vi "Create Framework Status.vi"(8 "error in (no error)":errorcluster, 11 "Framework Configuration":refnum<class "Framework Configuration.lvclass">) -> (0 "error out":errorcluster, 3 "Framework Status":refnum<class "Framework Status.lvclass">)   [LabVIEW 2021, in "DSF Core.lvlib" / "Framework Status.lvclass"]
uses:
  Framework Status.lvclass
  Configuration/Core/Framework/Framework Configuration.lvclass
  Status/Status Data.ctl
  <vilib>/NI/Memory Manager/Classes/Pointer/Pointer.lvclass/Pointer.ctl
  Framework Status.lvclass/Framework Status.ctl
  <vilib>/NI/Memory Manager/Classes/Pointer/Allocate.vi
  Status/Status Size.vi
  Status/Write Status 1D.vi
  <vilib>/NI/Memory Manager/Classes/Pointer/Set Address.vi
  <vilib>/NI/Memory Manager/Classes/Pointer/Set Size.vi
  <vilib>/NI/Memory Manager/Classes/Pointer/Set Internal.vi
  <vilib>/NI/Memory Manager/Classes/Pointer/Get Address.vi
  <vilib>/NI/Memory Manager/Classes/Pointer/Check Size.vi
  <vilib>/NI/Memory Manager/Classes/Pointer/Check Null Pointer.vi
  <vilib>/NI/Memory Manager/Classes/Pointer/Errors.vi
  <vilib>/NI/Memory Manager/Classes/Pointer/Out of Bounds.vi
  <vilib>/NI/Memory Manager/Classes/Pointer/Get Size.vi
  <vilib>/NI/Memory Manager/Classes/Pointer/Null Pointer.vi
  <vilib>/NI/Memory Manager/Classes/Pointer/Is Null.vi
  <vilib>/NI/Memory Manager/VIs/Write String to Source.vi
  <vilib>/NI/Memory Manager/Classes/Pointer/Write Pointer Size to Error.vi
  <vilib>/NI/Memory Manager/Classes/Pointer/Create Error.vi
  <vilib>/NI/Memory Manager/VIs/Write Numeric to Source.vi
  <vilib>/NI/Memory Manager/VIs/Write Numeric Scalar to Source (Base10 U64).vi
  <vilib>/NI/Memory Manager/VIs/New Error Cluster.vi
  <vilib>/NI/Memory Manager/VIs/New Error Cluster (512B).vi
  <vilib>/NI/Memory Manager/VIs/Set Error Status.vi
  <vilib>/NI/Memory Manager/VIs/Set Error Code.vi
  <vilib>/NI/Memory Manager/VIs/Set Error Source.vi
  <vilib>/NI/Memory Manager/Constants/Constants.vi
  <vilib>/NI/Memory Manager/Constants/Library Name.vi
  <vilib>/NI/Memory Manager/Classes/Pointer/Pointer Error Info.vi
  <vilib>/NI/Memory Manager/Constants/Pointer Class Name.vi
  Status/Status Pointer.lvclass
  C:/Program Files/National Instruments/LabVIEW 2021/vi.lib/NI/Memory Manager/Classes/Pointer/Pointer.lvclass
  Configuration/Core/Plugin/Plugin Configuration.lvclass
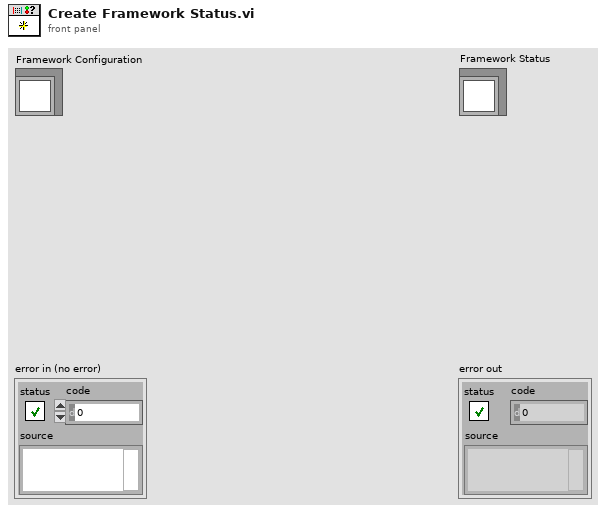
[diagram p1: front panel]
types:
  T1 = typedef "DSF Core.lvlib/Status Pointer.lvclass/Status Data.ctl" = cluster{"duration":u64, "period":u64, "iteration":u64, "late count":u64}
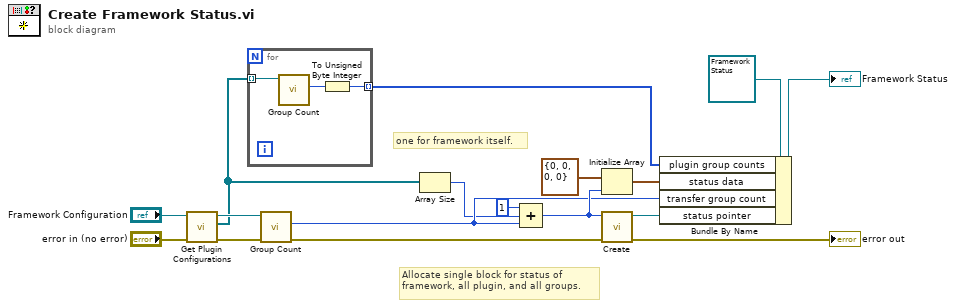
[diagram p0: block diagram]
diagram:
  # "Allocate single block for status of framework, all plugin, and all groups."
  # "one for framework itself."
  n1 = call "Get Plugin Configurations.vi"("error in (no error)"="error in (no error)", "Framework Configuration in"="Framework Configuration") -> ("error out"=w6:errorcluster, "Plugin Configurations"=w2:refnum<class "Plugin Configuration.lvclass">[], "Framework Configuration out"=w5:refnum<class "Framework Configuration.lvclass">)  [unwired: 7 in]
  n2 = for {
    tunnel: w2 -> [w20] mode=indexing
    tunnel: [w19] -> w9 mode=indexing
    n3 = call-dynamic "Group Count.vi"("Plugin Configuration in"=w20) -> ("group count"=w18:i32)  [unwired: 8 in, 2 out]
    n4 = To Unsigned Byte Integer(number=w18) -> (unsigned 8bit integer=w19:u8)
  }
  n5 = call-dynamic "Group Count.vi"("error in (no error)"=w6, "Framework Configuration in"=w5) -> ("error out"=w4:errorcluster, "group count"=w3:i32)  [unwired: 7 in, 1 out]
  n6 = Array Size(array=w2) -> (size(s)=w1:i32)
  n7 = Compound Arithmetic op=ADD(1 ("value"), w1, w3) -> (w11:i32)
  n8 = Initialize Array(T1 {"duration"=0, "period"=0, "iteration"=0, "late count"=0} ("status data"), w11) -> (w10:T1[])
  n9 = call "Create.vi"("error in (no error)"=w4, "count (1)"=w11) -> ("error out"=→"error out":errorcluster, "status pointer"=w14:refnum<class "Status Pointer.lvclass">)  [unwired: 8 in]
  n10 = Bundle By Name(cluster=refnum<class "Framework Status.lvclass"> refnum ("Framework Status in"), "plugin group counts"=w9, "status data"=w10, "transfer group count"=w3, "status pointer"=w14) -> (→"Framework Status":refnum<class "Framework Status.lvclass">)
